vi "optogeneticsSelectFromList.vi"(0 "XYZ":i32[][](array[numeric]), 1 "targetIndices (:-separated, -1 for all)":string="0") -> (2 "X":i32[](array[numeric]), 3 "Y":i32[](array[numeric]), 4 "Z":i32[](array[numeric]))   [LabVIEW 2017]
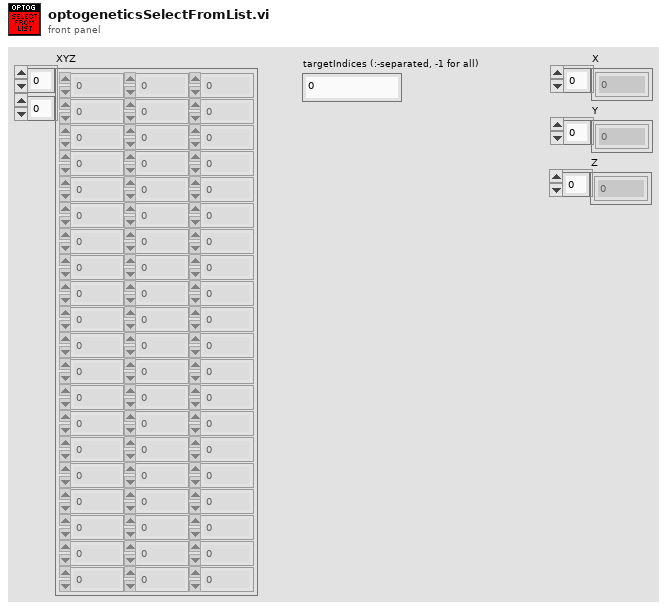
[diagram p1: front panel]
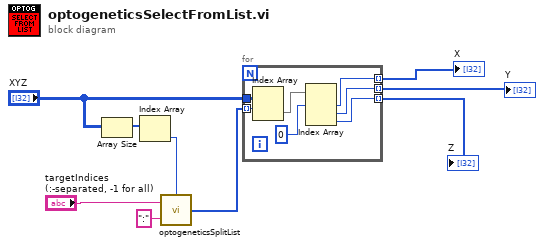
[diagram p0: block diagram]
diagram:
  n1 = Array Size(array="XYZ") -> (size(s)=w4:i32[])
  n2 = Index Array(array=w4) -> (element=w2:i32)  [unwired: 1 in]
  n3 = call "optogeneticsSplitList.vi"("max"=w2, "delimiter"=":", "list"="targetIndices (:-separated, -1 for all)") -> ("output"=w5:i32[])
  n4 = for {
    tunnel: "XYZ" -> [w16]
    tunnel: [w13] -> w9 mode=indexing
    tunnel: [w12] -> w8 mode=indexing
    tunnel: [w11] -> w7 mode=indexing
    tunnel: w5 -> [w10] mode=indexing
    n5 = Index Array(array=w16, index (row)=w10) -> (element=w15:i32[])  [unwired: 1 in]
    n6 = Index Array(array=w15, index #1=0 ("index")) -> (element #1=w13:i32, element #2=w12:i32, element #3=w11:i32)  [unwired: 2 in]
  }
  "X" <- w9
  "Y" <- w8
  "Z" <- w7
